vi "CalculateSinus.vi"(1 "As":dbl caption="Амплитуда сигнала, As", 2 "t, [s]":dbl=1.0 caption="Время t, [s]", 3 "f, [Hz]":dbl=1.0 caption="Частота сигнала f, [Hz]") -> (0 "Значение синуса":dbl)   [LabVIEW 2019]
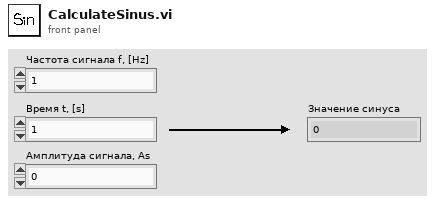
[diagram p1: front panel]
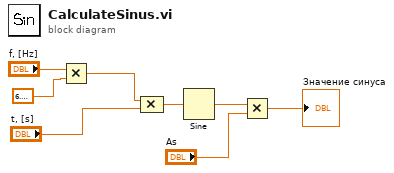
[diagram p0: block diagram]
diagram:
  n1 = Multiply(x="f, [Hz]", y=6.283185307179586) -> (x*y=w6:dbl)
  n2 = Compound Arithmetic op=MULTIPLY(w6, "t, [s]") -> (w4:dbl)
  n3 = Sine(x=w4) -> (sin(x)=w3:dbl)
  n4 = Multiply(x=w3, y="As") -> (x*y=→"Значение синуса":dbl)
